vi "obsitcle avoidance.vi"(8 "target y":i16, 9 "target x":i16, 11 "distance 3":fxp<+/-,32,16>[](array[numeric])) -> (0 "target y 2":i16, 1 "target x 2":i16, 4 "not done":bool=TRUE)   [LabVIEW 2014]
uses:
  Robot Global Data.vi
panel:
  in  "current y":i16
  in  "current x":i16
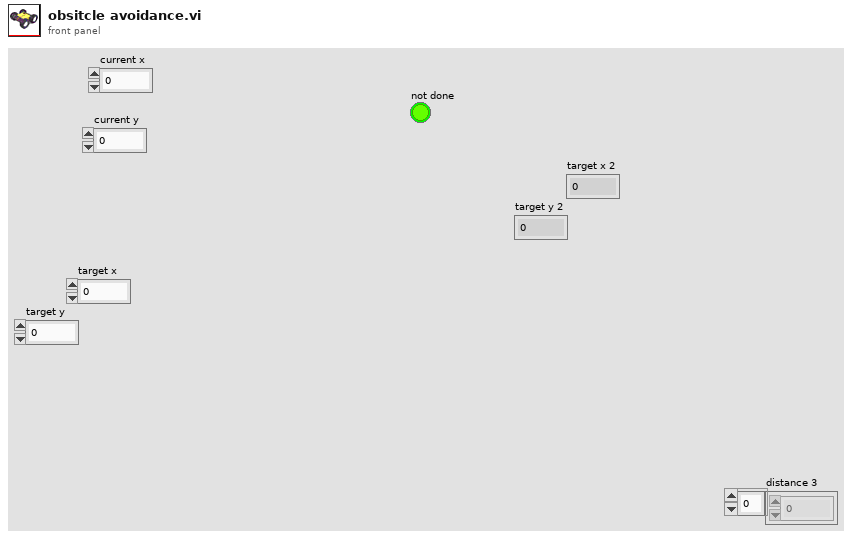
[diagram p1: front panel]
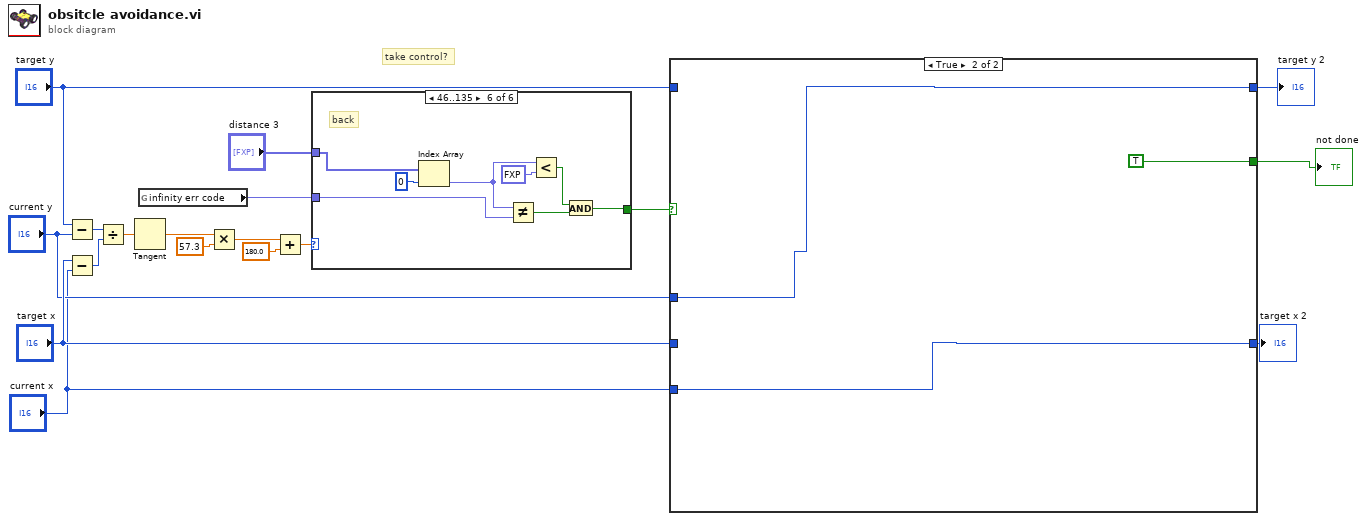
[diagram p0: block diagram]
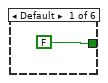
[diagram p2: hidden frame]
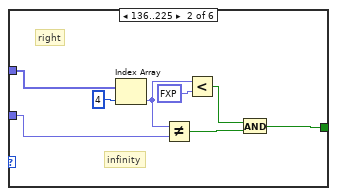
[diagram p3: hidden frame]
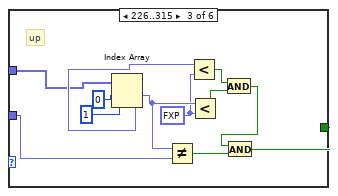
[diagram p4: hidden frame]
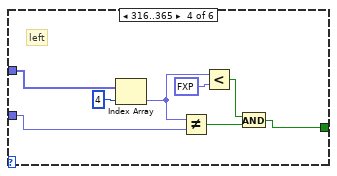
[diagram p5: hidden frame]
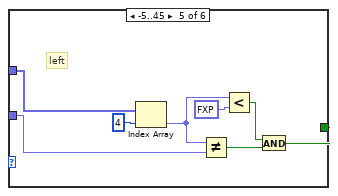
[diagram p6: hidden frame]
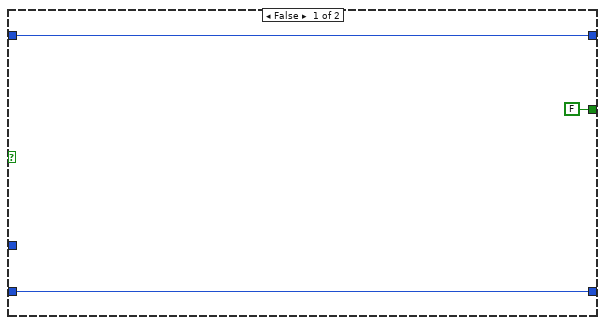
[diagram p7: hidden frame]
diagram:
  # "take control?"
  n1 = Subtract(x="target y", y="current y") -> (x-y=w14:i16)
  n2 = Subtract(x="target x", y="current x") -> (x-y=w13:i16)
  n3 = Divide(x=w14, y=w13) -> (x/y=w12:dbl)
  n4 = Tangent(1:w12) -> (0:w11:dbl)
  n5 = global read "Robot Global Data.vi" "infinity err code"() -> (w1:fxp<+/-,32,16>)
  n6 = Multiply(x=w11, y=57.3) -> (x*y=w9:dbl)
  n7 = Add(x=w9, y=180.0) -> (x+y=w6:dbl)
  n8 = case shown="46..135" w6 {
    tunnel: [FALSE w22 w36 w42 w50 w58] -> w7
    tunnel: "distance 3" -> [_ w21 w29 w41 w49 w57]
    tunnel: w1 -> [_ w20 w28 w40 w48 w56]
    frame Default {
    }
    frame 136..225 {
      # "infinity"
      # "right"
      n9 = Index Array(array=w21, index=4) -> (element=w23:fxp<+/-,32,16>)
      n10 = Not Equal?(x=w23, y=w20) -> (x != y?=w24:bool)
      n11 = Less?(x=w23, y=fxp<+/-,32,16> 160.0) -> (x < y?=w25:bool)
      n12 = And(x=w25, y=w24) -> (x .and. y?=w22:bool)
    }
    frame 226..315 {
      w33 = fxp<+/-,32,16> 160.0 ("y")
      # "up"
      n13 = Index Array(array=w29, index #1=0 ("index"), index #2=1 ("index")) -> (element #1=w37:fxp<+/-,32,16>, element #2=w34:fxp<+/-,32,16>)
      n14 = Not Equal?(x=w37, y=w28) -> (x != y?=w38:bool)
      n15 = Less?(x=w34, y=w33) -> (x < y?=w32:bool)
      n16 = Less?(x=w37, y=w33) -> (x < y?=w31:bool)
      n17 = And(x=w32, y=w31) -> (x .and. y?=w30:bool)
      n18 = And(x=w30, y=w38) -> (x .and. y?=w36:bool)
    }
    frame 316..365 {
      # "left"
      n19 = Index Array(array=w41, index=4) -> (element=w43:fxp<+/-,32,16>)
      n20 = Not Equal?(x=w43, y=w40) -> (x != y?=w44:bool)
      n21 = Less?(x=w43, y=fxp<+/-,32,16> 160.0) -> (x < y?=w45:bool)
      n22 = And(x=w45, y=w44) -> (x .and. y?=w42:bool)
    }
    frame -5..45 {
      # "left"
      n23 = Index Array(array=w49, index=4) -> (element=w51:fxp<+/-,32,16>)
      n24 = Not Equal?(x=w51, y=w48) -> (x != y?=w52:bool)
      n25 = Less?(x=w51, y=fxp<+/-,32,16> 160.0) -> (x < y?=w53:bool)
      n26 = And(x=w53, y=w52) -> (x .and. y?=w50:bool)
    }
    frame 46..135 {
      # "back"
      n27 = Index Array(array=w57, index=0) -> (element=w59:fxp<+/-,32,16>)
      n28 = Not Equal?(x=w59, y=w56) -> (x != y?=w60:bool)
      n29 = Less?(x=w59, y=fxp<+/-,32,16> 160.0) -> (x < y?=w61:bool)
      n30 = And(x=w61, y=w60) -> (x .and. y?=w58:bool)
    }
  }
  n31 = case shown="True" w7 {
    tunnel: "target x" -> [w66 _]
    tunnel: [w66 w68] -> w18
    tunnel: "target y" -> [w65 _]
    tunnel: [w65 w69] -> w17
    tunnel: "current y" -> [_ w69]
    tunnel: "current x" -> [_ w68]
    tunnel: [FALSE TRUE] -> w3
    frame False {
    }
    frame True {
    }
  }
  "target x 2" <- w18
  "target y 2" <- w17
  "not done" <- w3
